vi "Flush Data to Log File.vi"(8 "error in (no error)":errorcluster, 10 "Data Queue":T1, 11 "Logging Configuration":T2) -> (0 "error out":errorcluster)   [LabVIEW 2018, in "Logging.lvlib"]
doc: "Flush the data queue of any pending data and write it to the log file. Close the TDMS file reference."
uses:
  Logging.lvlib
  Logging Configuration.ctl
  Controls/Data Queue.ctl
  library/Datalogger LLB/Data Record Control.ctl
  library/Datalogger LLB/Datalogger.lvclass
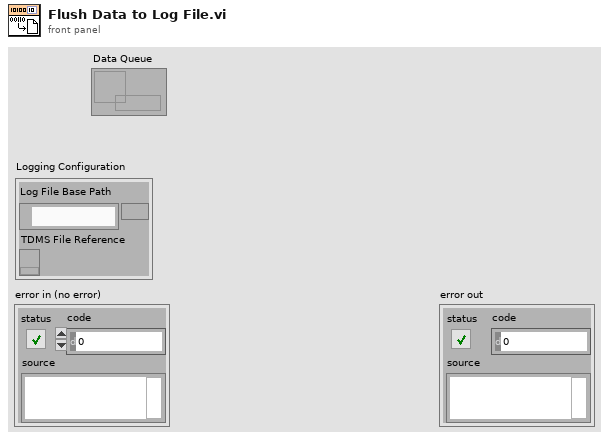
[diagram p1: front panel]
types:
  T1 = typedef "Data Queue.ctl" = refnum<queue>
  T2 = typedef "Logging.lvlib/Logging Configuration.ctl" = cluster{"Log File Base Path":path, "TDMS File Reference":refnum<k34>}
  T3 = typedef "Datalogger.lvlib/Datalogger.lvclass/Data Record Control.ctl" = cluster{"Timestamp":string, "Sensor Name":string, "Data (string)":string, "Units":string}
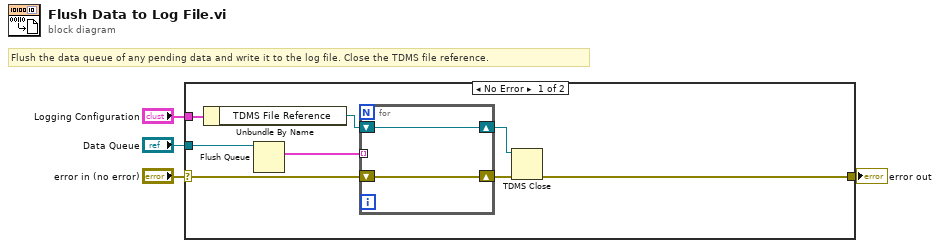
[diagram p0: block diagram]
diagram:
  # "Flush the data queue of any pending data and write it to the log file. Close the TDMS file reference."
  n1 = case shown="No Error" "error in (no error)" {
    selector: "error in (no error)" -> [w5 w15]
    tunnel: "Data Queue" -> [w8 _]
    tunnel: "Logging Configuration" -> [w7 _]
    tunnel: [w6 w15] -> w3
    frame No Error {
      n2 = Unbundle By Name(w7) -> ("TDMS File Reference"=w9:refnum<k34>)
      n3 = Flush Queue(queue=w8) -> (remaining elements=w12:T3[])  [unwired: 1 in, 2 out]
      n4 = for {
        shift-right: [w13] -> w10
        shift-left: w9 -> [w13]
        shift-right: [w14] -> w11
        shift-left: w5 -> [w14]
        tunnel: w12 -> [_] mode=indexing
      }
      n5 = TDMS Close(8:w11, 11:w10) -> (0:w6:errorcluster)  [unwired: 1 out]
    }
    frame Error {
    }
  }
  "error out" <- w3
